vi "SetTimeSampleTrigger.vi"(0 "controller in":refnum<k24>, 5 "period":dbl=1.0, 7 "units":i32(ring)=2 items=["Seconds", "Minutes", "Milliseconds", "Microseconds"], 11 "error in (no error)":errorcluster) -> (4 "controller out":refnum<k24>, 15 "error out":errorcluster)   [LabVIEW 2010]
uses:
  c:/aerotech/controller/dev/A3200/pc/labview/2010/bin/Aerotech.A3200.dll
  bin/Aerotech.A3200.dll
  c:/aerotech/controller/dev/A3200/pc/labview/2010/bin/Aerotech.A3200.LabVIEW.dll
  bin/Aerotech.A3200.LabVIEW.dll
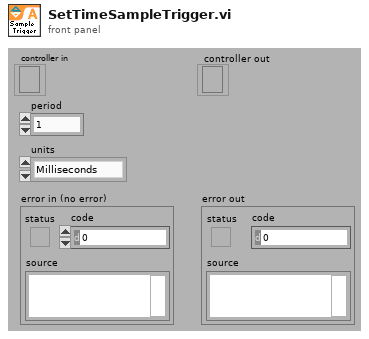
[diagram p1: front panel]
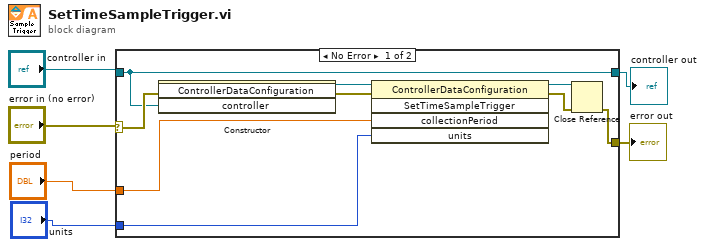
[diagram p0: block diagram]
diagram:
  n1 = case shown="No Error" "error in (no error)" {
    selector: "error in (no error)" -> [w14 w17]
    tunnel: "controller in" -> [w13 w16]
    tunnel: "period" -> [w11 _]
    tunnel: [w15 w17] -> w1
    tunnel: [w13 w16] -> w2
    tunnel: "units" -> [w10 _]
    frame No Error {
      n2 = constructor class="ControllerDataConfiguration"(error in=w14, "controller"=w13) -> (reference out=w7:refnum<k24>, error out=w12:errorcluster)  [unwired: 2 in, 2 out]
      n3 = invoke class="ControllerDataConfiguration" method="SetTimeSampleTrigger"(reference=w7, error in=w12, "collectionPeriod"=w11, "units"=w10) -> (reference out=w9:refnum<k24>, error out=w8:errorcluster)  [unwired: 1 in, 3 out]
      n4 = Close Reference(reference=w9, error in (no error)=w8) -> (error out=w15:errorcluster)
    }
    frame Error {
    }
  }
  "controller out" <- w2
  "error out" <- w1
